vi "Add Linked List.vi"(6 "Insertion Index":i32=-1, 7 "Parent ID":string, 8 "error in (no error)":errorcluster, 9 "Unique ID":string, 10 "Name":string, 11 "Linked List in":refnum<class "Linked List.lvclass">) -> (0 "error out":errorcluster, 1 "Replaced?":bool, 3 "Linked List out":refnum<class "Linked List.lvclass">, 5 "Unique ID out":string)   [LabVIEW 2020, in "Linked Lists.lvlib" / "Linked List.lvclass"]
uses:
  <vilib>/gpm_packages/@cs/linked-list/Source/Linked List/Linked List/Linked List.lvclass
  <vilib>/gpm_packages/@cs/linked-list/Source/Linked List/Linked List Definition/Linked List Definition.lvclass
  <vilib>/gpm_packages/@cs/linked-list/Source/Linked List/Linked List/Linked List.lvclass/Linked List.ctl
  <vilib>/gpm_packages/@cs/lookup-table/Source/LookupTable/LookupTable.lvclass/LookupTable.ctl
  40d841d8-d163-42b6-a4b6-3ac5bb61525b.vi
  d324b322-4ce1-447a-8a13-53545e93ae15.vi
  fc812a40-f069-411d-b258-bda0560e3025.vi
  40d81e3a-01e1-4f52-8a05-44961c959c9c.vi
  9e2f1362-8d6d-4e4b-9bcd-7dc2d0ef4263.vi
  5f0b58f1-0d62-406d-a6e2-3f028f25fa47.vi
  6f57e330-4f2f-4e28-88d0-f1aa37c4842d.vi
  <vilib>/gpm_packages/@cs/lookup-table/Source/LookupTable/Read Table Reference.vi
  40d841d8-d163-42b6-a4b6-3ac5bb61525b.vi/5a7267ad-595e-4610-9ac2-8bef780848ff.vi
  d324b322-4ce1-447a-8a13-53545e93ae15.vi/5a7267ad-595e-4610-9ac2-8bef780848ff.vi
  fc812a40-f069-411d-b258-bda0560e3025.vi/527409de-c0d9-4f52-b5ac-fa7c64bbfe33.vi
  40d81e3a-01e1-4f52-8a05-44961c959c9c.vi/527409de-c0d9-4f52-b5ac-fa7c64bbfe33.vi
  9e2f1362-8d6d-4e4b-9bcd-7dc2d0ef4263.vi/527409de-c0d9-4f52-b5ac-fa7c64bbfe33.vi
  5f0b58f1-0d62-406d-a6e2-3f028f25fa47.vi/527409de-c0d9-4f52-b5ac-fa7c64bbfe33.vi
  6f57e330-4f2f-4e28-88d0-f1aa37c4842d.vi/527409de-c0d9-4f52-b5ac-fa7c64bbfe33.vi
  <vilib>/gpm_packages/@cs/lookup-table/Source/LookupTable/LookupTable.lvclass
  <vilib>/gpm_packages/@cs/linked-list/Source/Linked List/Linked List Header/Linked List Header.lvclass
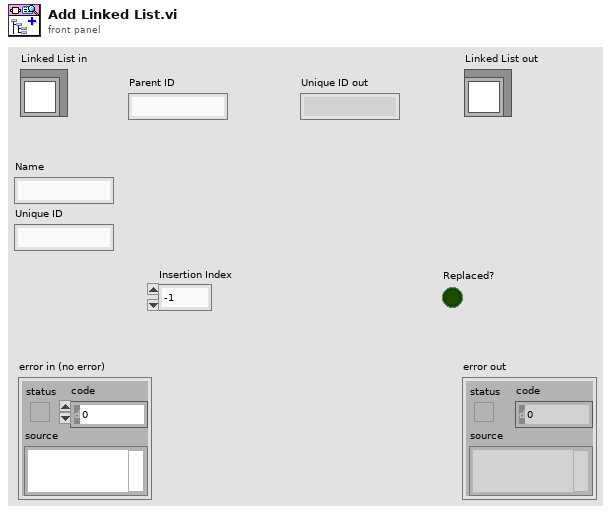
[diagram p1: front panel]
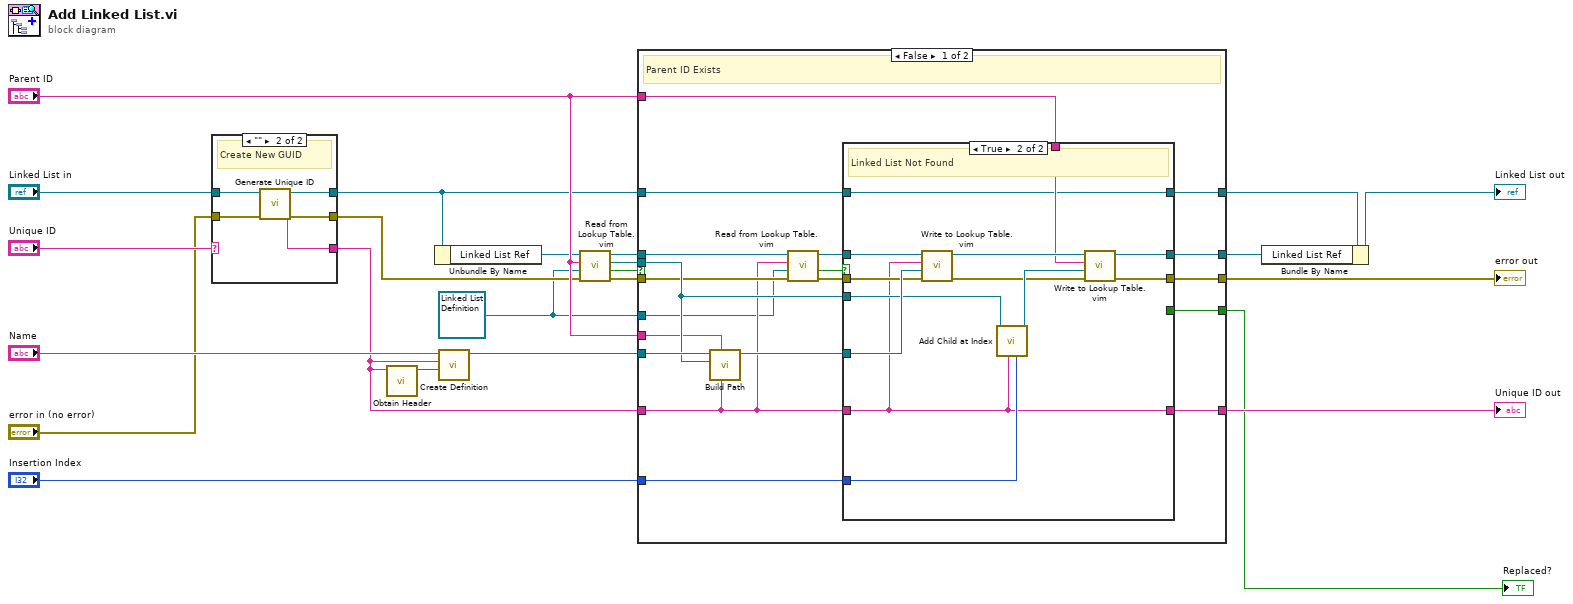
[diagram p0: block diagram]
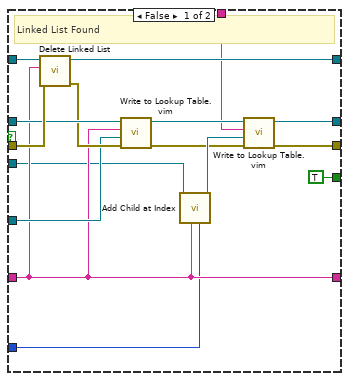
[diagram p2: hidden frame]
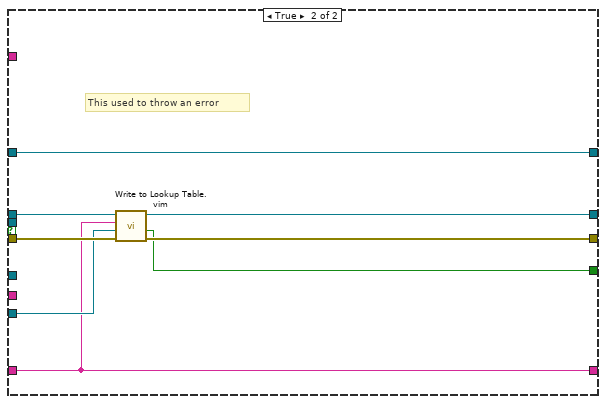
[diagram p3: hidden frame]
diagram:
  w1 = refnum<class "Linked List Definition.lvclass"> refnum ("Linked List.lvlib:Linked List Definition.lvclass")
  n1 = case shown="\"\"" "Unique ID" {
    selector: "Unique ID" -> [w26 _]
    tunnel: "Linked List in" -> [w25 w31]
    tunnel: [w26 w30] -> w11
    tunnel: [w25 w29] -> w7
    tunnel: "error in (no error)" -> [w24 w28]
    tunnel: [w24 w27] -> w5
    frame Default {
      # "Use existing GUID"
    }
    frame "" {
      # "Create New GUID"
      n2 = call <vilib>:"Generate Unique ID.vi"("error in (no error)"=w28, "Linked List in"=w31) -> ("error out"=w27:errorcluster, "ID"=w30:string, "Linked List out"=w29:refnum<class "Linked List.lvclass">)  [unwired: 7 in]
    }
  }
  n3 = call <vilib>:"Obtain Header.vi"("GUID"=w11) -> ("Linked List Header out"=w14:refnum<class "Linked List Header.lvclass">)  [unwired: 9 in, 1 out]
  n4 = Unbundle By Name(w7) -> ("Linked List Ref"=w13:refnum<data-value>)
  n5 = call <vilib>:"Create Definition.vi"("Header"=w14, "Unique ID"=w11, "Name"="Name") -> ("Linked List Definition out"=w12:refnum<class "Linked List Definition.lvclass">)  [unwired: 8 in]
  n6 = call "Read from Lookup Table.vim"("error in (no error)"=w5, "Type"=w1, "Item Name"="Parent ID", "LookupTable Reference"=w13) -> ("error out"=w4:errorcluster, "Not Found?"=w3:bool, "Value"=w8:refnum<class "Linked List Definition.lvclass">, "LookupTable Reference Out"=w9:refnum<data-value>)  [unwired: 4 in]
  n7 = case shown="False" w3 {
    tunnel: w12 -> [w50 w83]
    tunnel: w11 -> [w37 w82]
    tunnel: [w49 w85] -> w10
    tunnel: w9 -> [w41 w86]
    tunnel: "Insertion Index" -> [w47 _]
    tunnel: w8 -> [w46 _]
    tunnel: "Parent ID" -> [w45 _]
    tunnel: "Parent ID" -> [w44 _]
    tunnel: [w34 w87] -> w6
    tunnel: w7 -> [w35 w87]
    tunnel: w4 -> [w39 w84]
    tunnel: [w43 w81] -> w15
    tunnel: [w33 w82] -> w16
    tunnel: [w42 w80] -> w2
    tunnel: w1 -> [w36 _]
    frame False {
      # "Parent ID Exists"
      n8 = call <vilib>:"Build Path.vi"("Unique ID"=w37, "Parent ID"=w45, "Parent Definition"=w46, "Linked List Definition in"=w50) -> ("Linked List Definition out"=w48:refnum<class "Linked List Definition.lvclass">)  [unwired: 6 in, 1 out]
      n9 = call "Read from Lookup Table.vim"("error in (no error)"=w39, "Type"=w36, "Item Name"=w37, "LookupTable Reference"=w41) -> ("error out"=w38:errorcluster, "Not Found?"=w32:bool, "LookupTable Reference Out"=w40:refnum<data-value>)  [unwired: 4 in, 1 out]
      n10 = case shown="True" w32 {
        tunnel: [w58 w79] -> w49
        tunnel: w48 -> [w57 w77]
        tunnel: w47 -> [w55 w76]
        tunnel: w46 -> [w54 w75]
        tunnel: w44 -> [w51 w73]
        tunnel: [w52 w71] -> w43
        tunnel: [TRUE ("Replaced?") _] -> w42
        tunnel: w40 -> [w60 w70]
        tunnel: w38 -> [w64 w69]
        tunnel: w37 -> [w56 w67]
        tunnel: [w65 w68] -> w34
        tunnel: w35 -> [w66 w68]
        tunnel: [w56 w67] -> w33
        frame False {
          # "Linked List Found"
          n11 = call-dynamic "Delete Linked List.vi"("error in (no error)"=w64, "Unique ID"=w56, "Linked List in"=w66) -> ("error out"=w59:errorcluster, "Linked List out"=w65:refnum<class "Linked List.lvclass">)  [unwired: 7 in]
          n12 = call "Write to Lookup Table.vim"("error in (no error)"=w59, "Item"=w57, "Item Name"=w56, "LookupTable Reference"=w60) -> ("error out"=w61:errorcluster, "LookupTable Reference Out"=w63:refnum<data-value>)  [unwired: 5 in, 1 out]
          n13 = call <vilib>:"Add Child at Index.vi"("Insertion Index"=w55, "Unique ID"=w56, "Linked List Definition in"=w54) -> ("Linked List Definition out"=w62:refnum<class "Linked List Definition.lvclass">)  [unwired: 8 in]
          n14 = call "Write to Lookup Table.vim"("error in (no error)"=w61, "Item"=w62, "Item Name"=w51, "LookupTable Reference"=w63) -> ("error out"=w52:errorcluster, "LookupTable Reference Out"=w58:refnum<data-value>)  [unwired: 5 in, 1 out]
        }
        frame True {
          # "Linked List Not Found"
          n15 = call "Write to Lookup Table.vim"("error in (no error)"=w69, "Item"=w77, "Item Name"=w67, "LookupTable Reference"=w70) -> ("error out"=w72:errorcluster, "LookupTable Reference Out"=w78:refnum<data-value>)  [unwired: 5 in, 1 out]
          n16 = call <vilib>:"Add Child at Index.vi"("Insertion Index"=w76, "Unique ID"=w67, "Linked List Definition in"=w75) -> ("Linked List Definition out"=w74:refnum<class "Linked List Definition.lvclass">)  [unwired: 8 in]
          n17 = call "Write to Lookup Table.vim"("error in (no error)"=w72, "Item"=w74, "Item Name"=w73, "LookupTable Reference"=w78) -> ("error out"=w71:errorcluster, "LookupTable Reference Out"=w79:refnum<data-value>)  [unwired: 5 in, 1 out]
        }
      }
    }
    frame True {
      # "This used to throw an error"
      n18 = call "Write to Lookup Table.vim"("error in (no error)"=w84, "Item"=w83, "Item Name"=w82, "LookupTable Reference"=w86) -> ("error out"=w81:errorcluster, "Replaced?"=w80:bool, "LookupTable Reference Out"=w85:refnum<data-value>)  [unwired: 5 in]
    }
  }
  "error out" <- w15
  "Unique ID out" <- w16
  "Replaced?" <- w2
  n19 = Bundle By Name(cluster=w6, "Linked List Ref"=w10) -> (→"Linked List out":refnum<class "Linked List.lvclass">)
